vi "selectionen accelerometre etmagneticsensrnsor.vi"(11 "Boolean":bool) -> (2 "address":i8)   [LabVIEW 2019]
uses:
  <vilib>/rvi/Emulation/niFpgaSctlEmulationGetInTimedLoop.vi
  <vilib>/rvi/Emulation/niFpgaProcessEmulError.vi
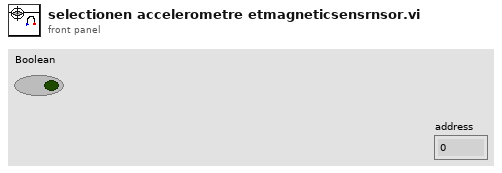
[diagram p1: front panel]
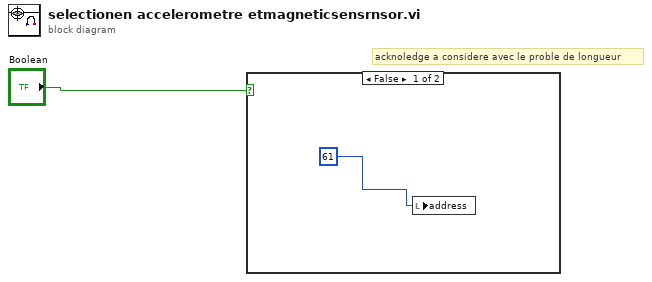
[diagram p0: block diagram]
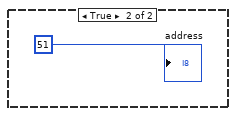
[diagram p2: hidden frame]
diagram:
  # "acknoledge a considere avec le proble de longueur"
  n1 = case shown="False" "Boolean" {
    frame False {
      n2 = local write "address"(i8 61) -> ()
    }
    frame True {
      "address" <- i8 51
    }
  }
